vi "Servidor - Fabrica.vi"() -> ()   [LabVIEW 2018]
doc: "Demonstrates how to establish multiple connections and place them in a queue to be serviced. As connections are made, it sends the current date and time via TCP to all Client VIs that connect to it.\n\nThis VI has two parts -- a loop that listens for each client to connect, and a loop that sends the date and time to each connection in the queue.\n\n<B>Note:</B> Use this VI with Multiple Connections - Client 1.vi and Multiple Connections - Client 2.vi."
uses:
  <vilib>/Utility/file.llb/Write Delimited Spreadsheet (string).vi
panel:
  out "Funcionamento:":string
  out "Alertas":u32(colorbox)
  in  "Histórico":i32(listbox)
  out "Thermometro\nForno":dbl(slide) scale=0.0..100.0
  out "Estoque\nProduto Final":dbl(slide) scale=0.0..2500.0
  out "Em Forno?":bool
  out "Misturando?":bool
  out "Solicitação\nMaterial B":dbl
  out "Solicitação\nMaterial A":dbl
  out "Estoque\nMaterial B":dbl(slide) scale=0.0..1200.0
  out "Estoque\nMaterial A":dbl(slide) scale=0.0..1200.0
  out "Mensagem da Produção:":string
  in  "Cliente a Receber os Dados:":string
  out "Cliente - Emissor de Dados:":string
  in  "Temperatura \nProdução [°C]":dbl(slide) scale=0.0..100.0
  out "Produto B":dbl
  in  "Produto A":dbl min=0.0 max=1000.0 step=1.0
  in  "Enviar Produção?":bool
  out "error out":errorcluster
  in  "RESETAR":bool
  in  "Iniciar\nProdução":bool
  in  "empty 3":refnum<k5>[](array[refnum])
  in  "stop":bool
  out "Protocolo de Envio:":string
  out "Conexões":i32
  in  "Porta":u16=6341
  out "IP da Máquina":string
  out "Mensagens":string
  in  "Enviar Todos":bool
  in  "listen halted":bool
  in  "empty":refnum<k5>[](array[refnum])
  # "SERVIDOR - FÁBRICA"
  # "Controle de Produção - Gerência"
  # "Kg"
  # "ON"
  # "ON"
  # "Kg"
  # "OFF"
  # "OFF"
  # "Levantamento de Dados da Produção"
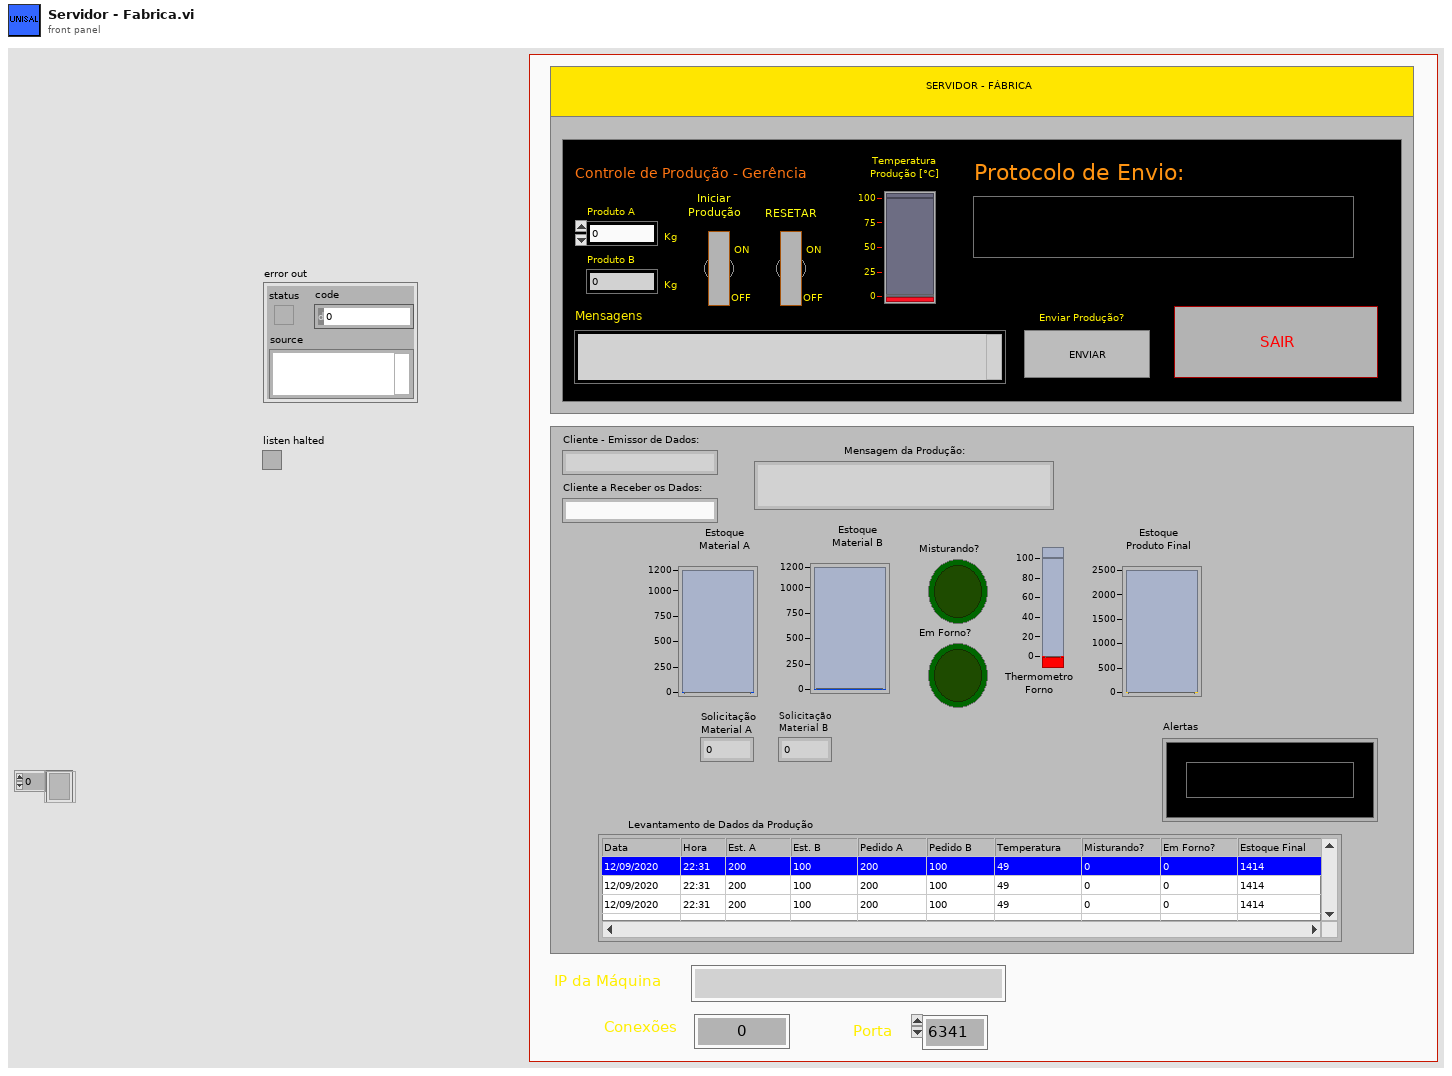
[diagram p1: front panel]
types:
  T1 = enum16{"Standard", "Buffered", "CRLF", "Immediate"}
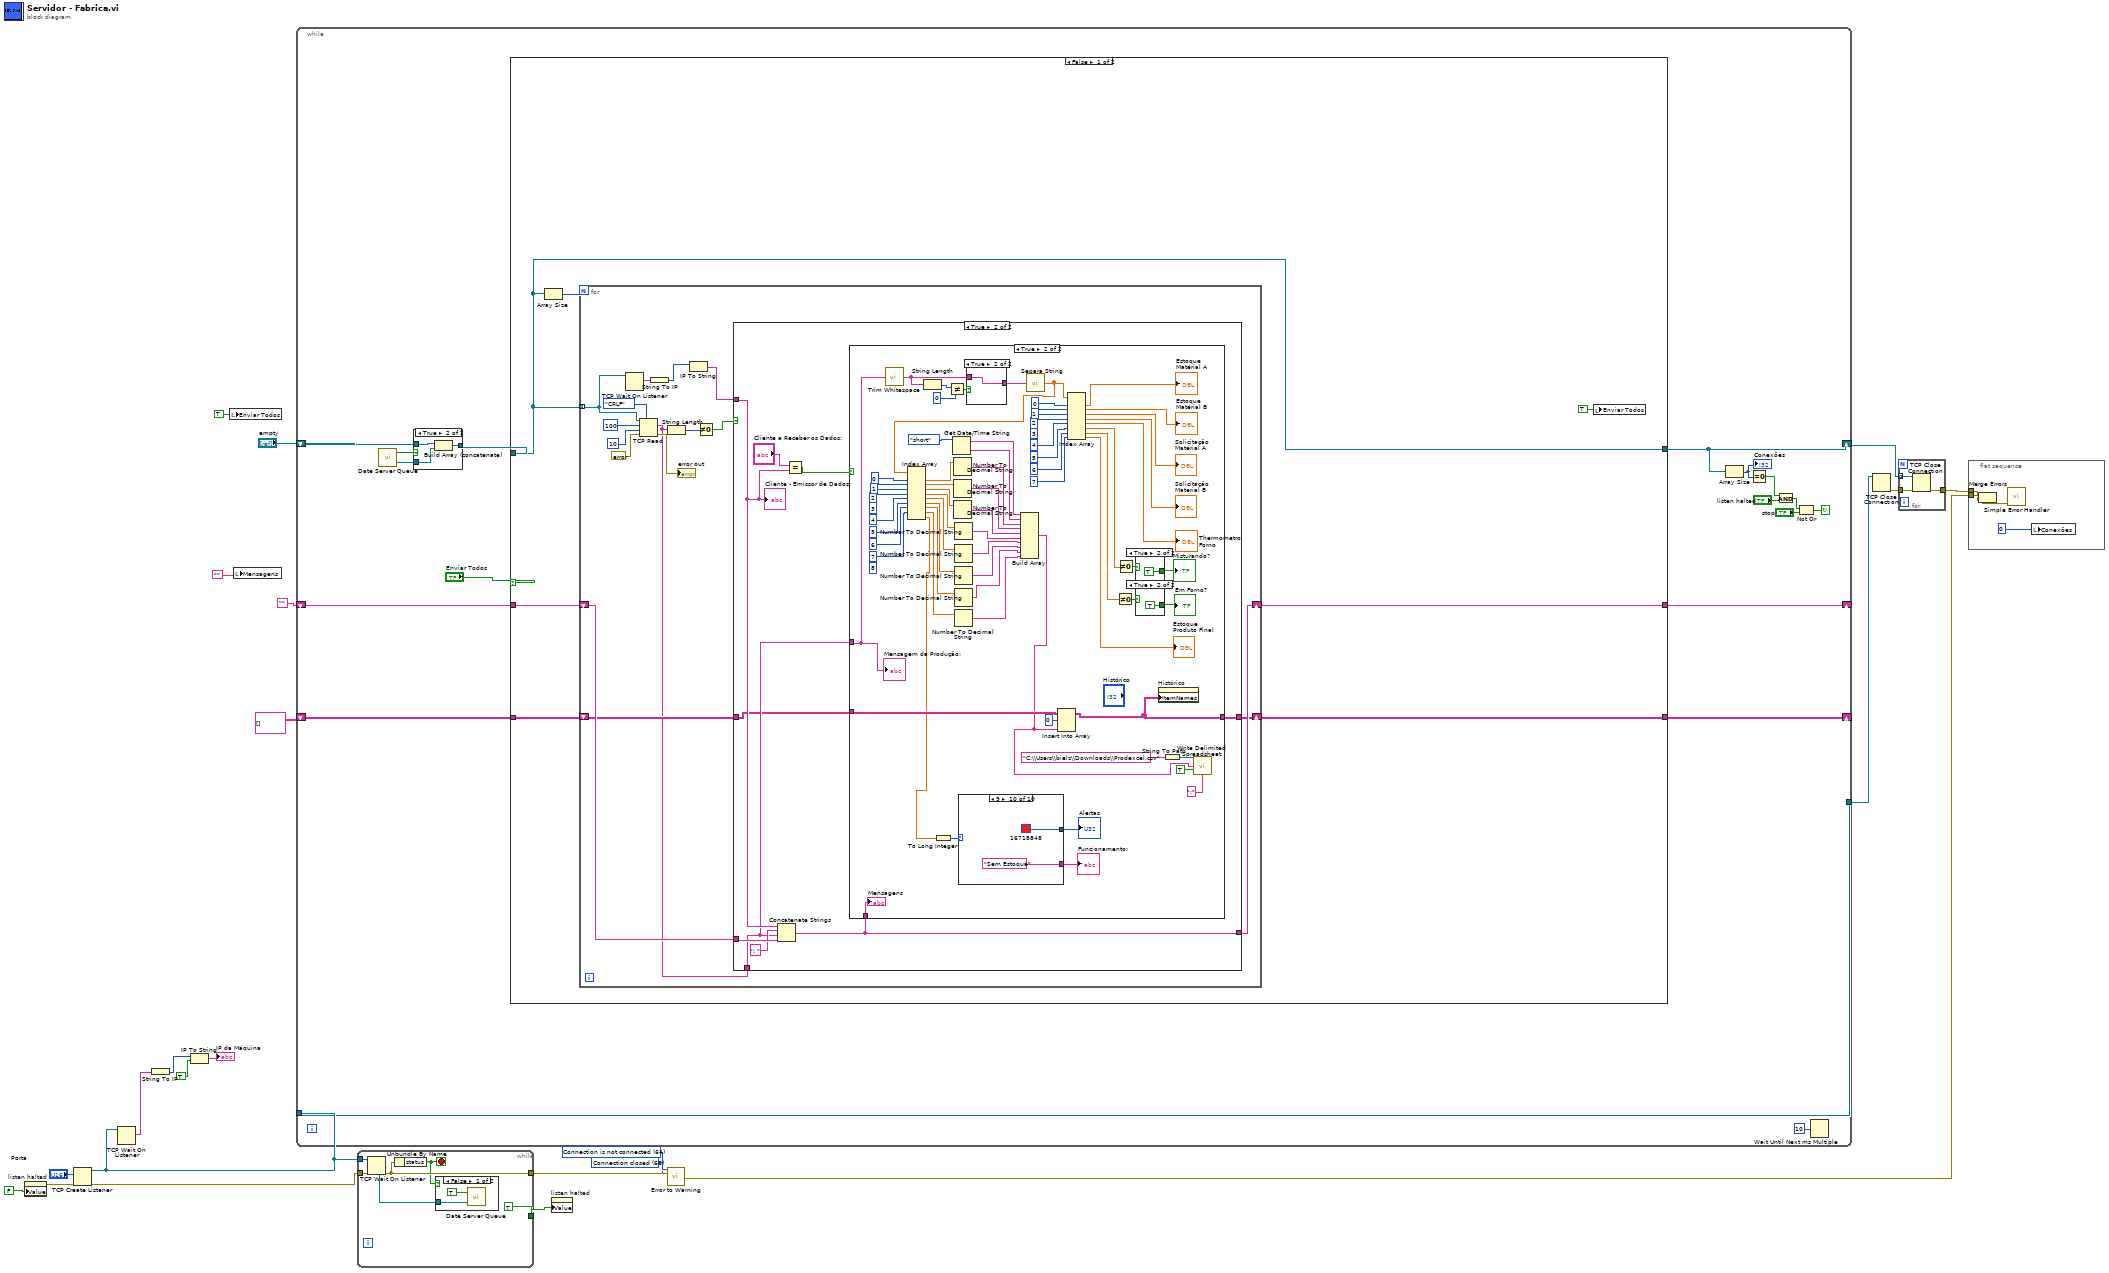
[diagram p0: block diagram]
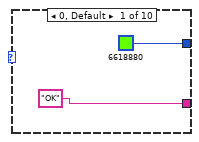
[diagram p4: hidden frame]
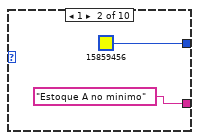
[diagram p5: hidden frame]
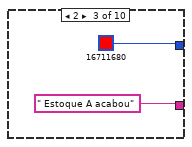
[diagram p6: hidden frame]
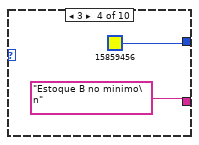
[diagram p7: hidden frame]
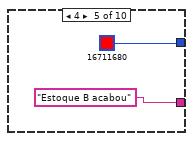
[diagram p8: hidden frame]
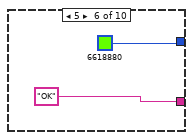
[diagram p9: hidden frame]
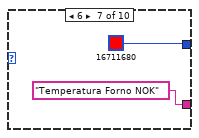
[diagram p10: hidden frame]
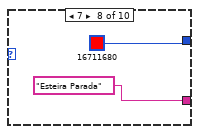
[diagram p11: hidden frame]
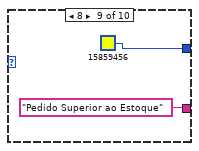
[diagram p12: hidden frame]
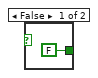
[diagram p13: hidden frame]
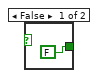
[diagram p14: hidden frame]
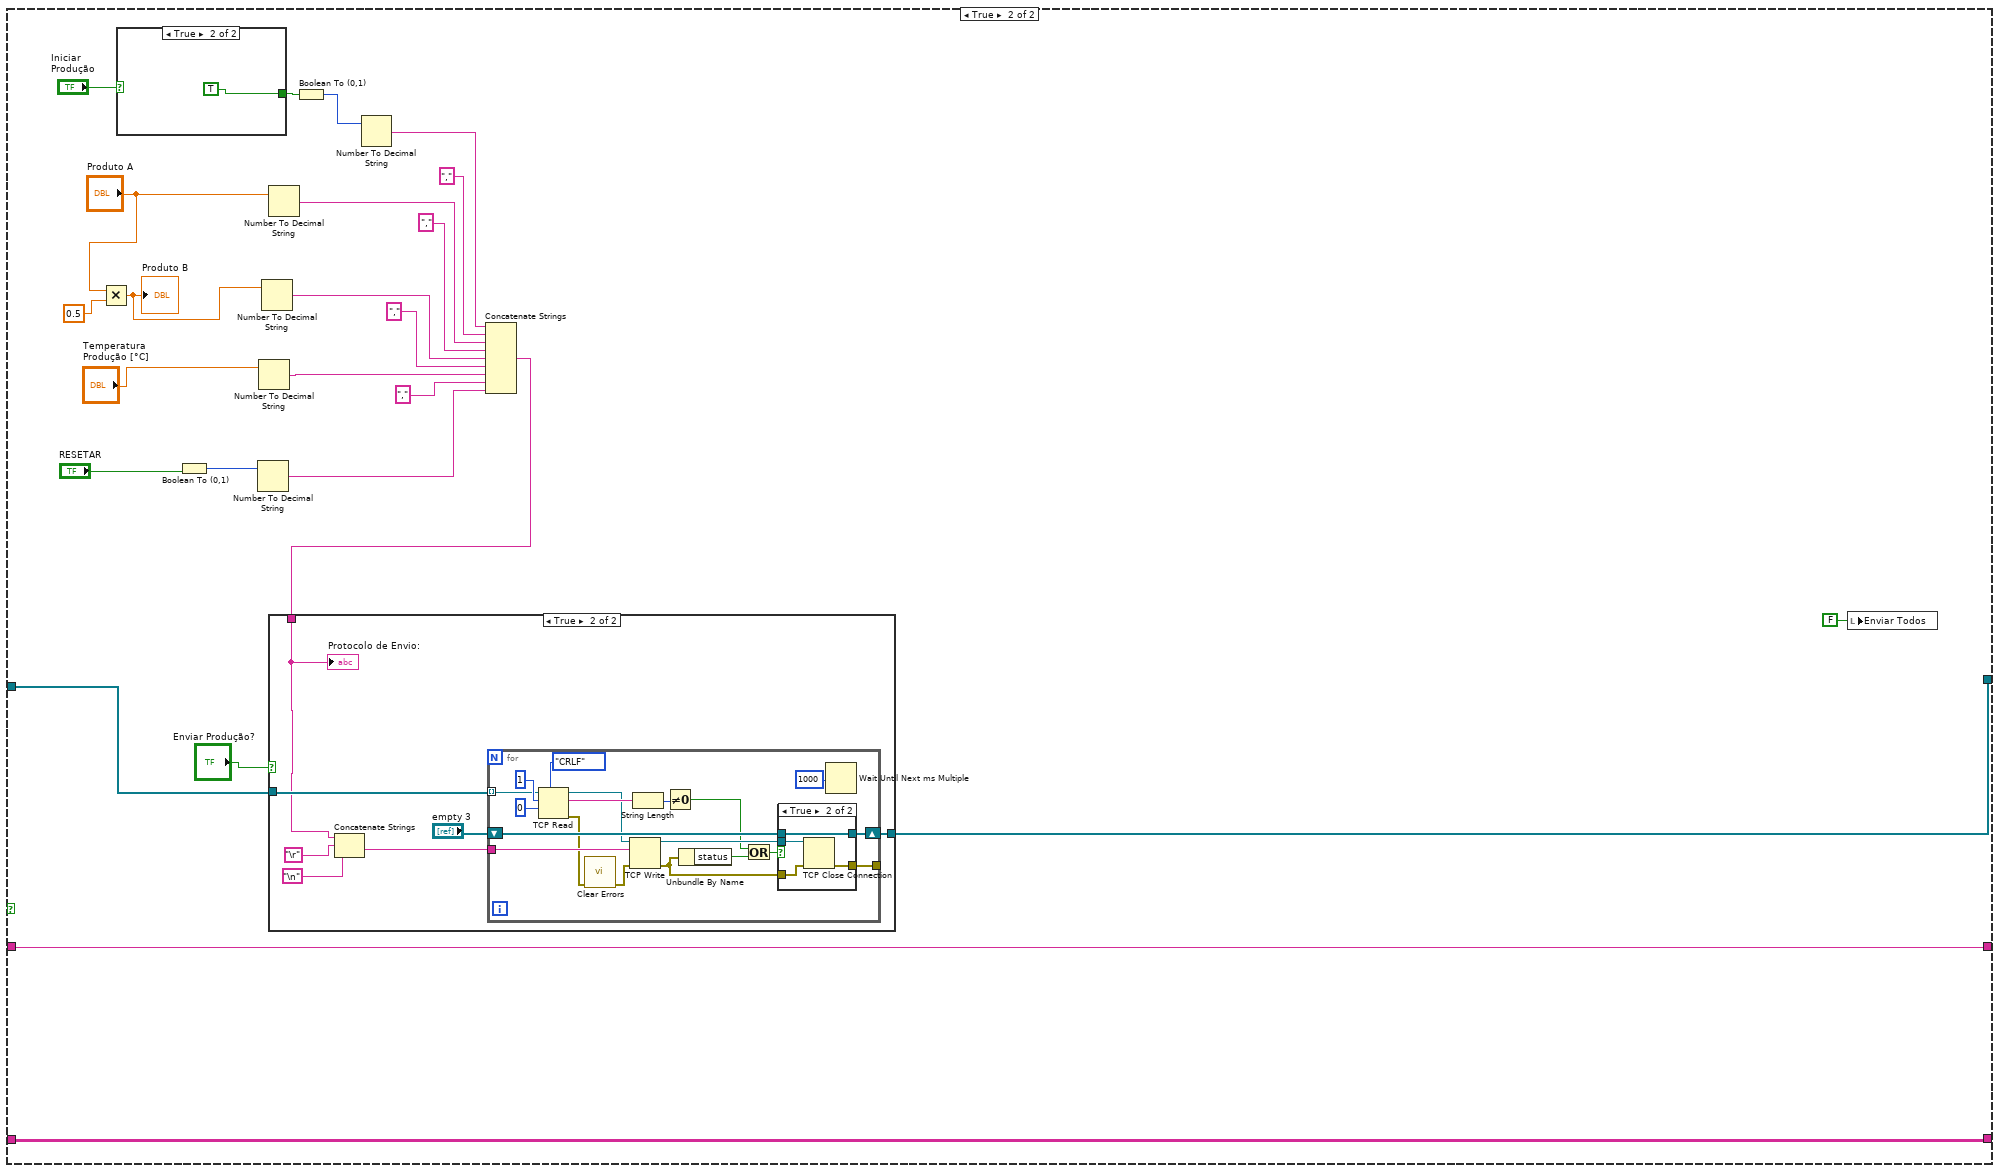
[diagram p16: hidden frame]
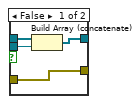
[diagram p18: hidden frame]
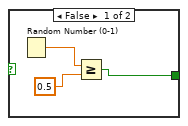
[diagram p19: hidden frame]
diagram:
  w16 = 66 items=["No Error", "Argument Error", "Memory Full", "Out of Zone", "End of File", "File Already Open", "Generic File IO Error", "File Not Found", "File Permission Error", "Disk Full", "Duplicate Path", "Too Many Files Open", "Not Enabled", "Resource File Not Found", "Cannot Add Resource", "Resource Not Found", "Image Not Found", "Image Memory Error", "Pen Does Not Exist", "Config Bad Type", "Config Token Not Found", "Config Parse Error", "Config Memory Error", "Bad External Code Format", "Bad External Code Offset", "External Code Not Present", "Null Window", "Destroy Window Mixup", "Null Menu", "Print Aborted", "Bad Print Record", "Print Driver Error", "Windows Error During Print", "Memory Error During Print", "Print Dialog Error", "Generic Print Error", "Invalid Device Refnum", "Device Not Found", "Device Parameter Error", "Device Unit Error", "Can't Open Device", "Device Call Aborted", "Generic Error", "Cancelled By User", "Object ID Too Low", "Object ID Too High", "Object Not In Heap", "Unknown Heap", "Bad DefProc ID", "DefProc Not In Table", "Message Out Of Range", "Null Method", "Unknown Message", "Manager Call Not Supported", "Bad address", "Connection In progress", "Connection timed out", "Connection is already in progress", "Network attribute not supported", "Network error", "Address in use", "System out of memory", "Connection aborted", "Connection refused", "Connection is not connected", "Connection is already connected", "Connection closed", "Initialize error (interapplication manager)", "Bad occurrence", "Wait on unbound occurrence handler", "Occurrence queue overflow", "Bad path", "Semaphore not signaled", "Unrecognized type (interapplication manager)"] ("2nd Error to Convert")
  w17 = 64 items=["No Error", "Argument Error", "Memory Full", "Out of Zone", "End of File", "File Already Open", "Generic File IO Error", "File Not Found", "File Permission Error", "Disk Full", "Duplicate Path", "Too Many Files Open", "Not Enabled", "Resource File Not Found", "Cannot Add Resource", "Resource Not Found", "Image Not Found", "Image Memory Error", "Pen Does Not Exist", "Config Bad Type", "Config Token Not Found", "Config Parse Error", "Config Memory Error", "Bad External Code Format", "Bad External Code Offset", "External Code Not Present", "Null Window", "Destroy Window Mixup", "Null Menu", "Print Aborted", "Bad Print Record", "Print Driver Error", "Windows Error During Print", "Memory Error During Print", "Print Dialog Error", "Generic Print Error", "Invalid Device Refnum", "Device Not Found", "Device Parameter Error", "Device Unit Error", "Can't Open Device", "Device Call Aborted", "Generic Error", "Cancelled By User", "Object ID Too Low", "Object ID Too High", "Object Not In Heap", "Unknown Heap", "Bad DefProc ID", "DefProc Not In Table", "Message Out Of Range", "Null Method", "Unknown Message", "Manager Call Not Supported", "Bad address", "Connection In progress", "Connection timed out", "Connection is already in progress", "Network attribute not supported", "Network error", "Address in use", "System out of memory", "Connection aborted", "Connection refused", "Connection is not connected", "Connection is already connected", "Connection closed", "Initialize error (interapplication manager)", "Bad occurrence", "Wait on unbound occurrence handler", "Occurrence queue overflow", "Bad path", "Semaphore not signaled", "Unrecognized type (interapplication manager)"] ("1st Error to Convert")
  n1 = property on="listen halted" class="Bool (strict)"("Value"=FALSE) -> (error out=w13:errorcluster)  [unwired: 2 in, 1 out]
  n2 = TCP Create Listener(8:w13, 10:"Porta") -> (0:w21:errorcluster, 3:w8:refnum<k5>)  [unwired: 3 in, 1 out]
  n3 = TCP Wait On Listener(11:w8) -> (2:w7:string)  [unwired: 3 in, 4 out]
  n4 = String To IP(1:w7) -> (0:w6:u32)
  n5 = IP To String(1:TRUE ("dot notation? (F)"), 2:w6) -> (0:→"IP da Máquina":string)
  n6 = local write "Enviar Todos"(TRUE ("Enviar Todos")) -> ()
  n7 = local write "Mensagens"("") -> ()
  n8 = while {
    shift-left: "empty" -> [w39]
    shift-right: [w31] -> w23
    tunnel: w8 -> [w32]
    tunnel: [w32] -> w20
    shift-right: [w27] -> _
    shift-left: "" -> [w28]
    shift-right: [w24] -> _
    shift-left: string[][] [] -> [w25]
    stop <- w34 continue-if-true
    n9 = call <vilib>:"Date Server Queue.vi"() -> ("value"=w41:refnum<k5>, "valid?"=w40:bool)  [unwired: 2 in]
    n10 = case shown="True" w40 {
      tunnel: w41 -> [_ w236]
      tunnel: w39 -> [w233 w235]
      tunnel: [w233 w234] -> w30
      frame False {
      }
      frame True {
        n11 = Build Array (concatenate)(w235, w236) -> (w234:refnum<k5>[])
      }
    }
    n12 = case shown="False" "Enviar Todos" {
      tunnel: w30 -> [w44 w193]
      tunnel: [w44 w192] -> w31
      tunnel: w28 -> [w47 w187]
      tunnel: [w46 w187] -> w27
      tunnel: w25 -> [w43 w169]
      tunnel: [w42 w169] -> w24
      frame False {
        n13 = Array Size(array=w44) -> (size(s)=w45:i32)
        n14 = for {
          N: w45 -> [_]
          tunnel: w44 -> [w53] mode=indexing
          shift-right: [w59] -> w46
          shift-left: w47 -> [w60]
          shift-right: [w50] -> w42
          shift-left: w43 -> [w51]
          n15 = TCP Wait On Listener(11:w53) -> (2:w55:string)  [unwired: 3 in, 4 out]
          n16 = TCP Read(connection ID=w53, bytes to read=100, error in (no error)=errorcluster {"status"=FALSE, "code"=0, "source"=""}, 7:T1."CRLF" ("mode (standard)"), 9:10 ("timeout ms (25000)")) -> (data out=w49:string, error out=→"error out":errorcluster)  [unwired: 1 out]
          n17 = String To IP(1:w55) -> (0:w54:u32)
          n18 = String Length(string=w49) -> (length=w63:i32)
          n19 = IP To String(2:w54) -> (0:w52:string)  [unwired: 1 in]
          n20 = Not Equal To 0?(x=w63) -> (x != 0?=w62:bool)
          n21 = case shown="True" w62 {
            tunnel: w49 -> [_ w70]
            tunnel: w60 -> [w66 w75]
            tunnel: [w66 w71] -> w59
            tunnel: w52 -> [_ w73]
            tunnel: w51 -> [w65 w69]
            tunnel: [w65 w68] -> w50
            frame False {
            }
            frame True {
              n22 = Concatenate Strings(w73, ": ", w70, w75) -> (w71:string)
              n23 = Equal?(x="Cliente a Receber os Dados:", y=w73) -> (x = y?=w67:bool)
              n24 = case shown="True" w67 {
                tunnel: w71 -> [_ w143]
                tunnel: w70 -> [_ w132]
                tunnel: w69 -> [w76 w87]
                tunnel: [w76 w86] -> w68
                frame False {
                }
                frame True {
                  (unwired) 8
                  n25 = call <vilib>:"Trim Whitespace.vi"("string"=w132) -> ("trimmed string"=w135:string)  [unwired: 1 in]
                  n26 = String Length(string=w135) -> (length=w134:i32)
                  n27 = Not Equal?(x=w134, y=0) -> (x != y?=w137:bool)
                  n28 = Get Date/Time String(date format (0)=enum16{"short", "long", "abbreviated"}."short") -> (date string=w98:string, time string=w97:string)  [unwired: 2 in]
                  n29 = case shown="True" w137 {
                    tunnel: [_ w168] -> w136
                    tunnel: w135 -> [_ w168]
                    frame False {
                    }
                    frame True {
                    }
                  }
                  n30 = call "Separa String.vi"("TEXTO DE ENTRADA"=w136) -> ("VETOR DE SAIDA"=w108:dbl[])
                  n31 = Index Array(array=w108, index #1=0 ("index"), index #2=1 ("index"), index #3=2 ("index"), index #4=3 ("index"), index #5=4 ("index"), index #6=5, index #7=6, index #8=7) -> (element #1=w106:dbl, element #2=w105:dbl, element #3=w104:dbl, element #4=w103:dbl, element #5=w102:dbl, element #6=w101:dbl, element #7=w100:dbl, element #8=w99:dbl, element #9=w77:dbl)  [unwired: 1 in]
                  n32 = To Long Integer(number=w77) -> (32bit integer=w78:i32)
                  n33 = Number To Decimal String(number=w106) -> (decimal integer string=w96:string)  [unwired: 1 in]
                  n34 = Number To Decimal String(number=w105) -> (decimal integer string=w95:string)  [unwired: 1 in]
                  n35 = Number To Decimal String(number=w104) -> (decimal integer string=w94:string)  [unwired: 1 in]
                  n36 = Number To Decimal String(number=w103) -> (decimal integer string=w93:string)  [unwired: 1 in]
                  n37 = Number To Decimal String(number=w102) -> (decimal integer string=w92:string)  [unwired: 1 in]
                  n38 = Number To Decimal String(number=w101) -> (decimal integer string=w91:string)  [unwired: 1 in]
                  n39 = Number To Decimal String(number=w100) -> (decimal integer string=w90:string)  [unwired: 1 in]
                  n40 = Number To Decimal String(number=w99) -> (decimal integer string=w89:string)  [unwired: 1 in]
                  n41 = case shown="9" w78 {
                    tunnel: ["OK" "Estoque A no minimo" " Estoque A acabou" "Estoque B no minimo\n" "Estoque B acabou" "OK" "Temperatura Forno NOK" "Esteira Parada" "Pedido Superior ao Estoque" "Sem Estoque"] -> w80
                    tunnel: [u32 6618880 ("Pedido") u32 15859456 ("Pedido") u32 16711680 ("Pedido") u32 15859456 ("Pedido") u32 16711680 ("Pedido") u32 6618880 ("Pedido") u32 16711680 ("Pedido") u32 16711680 ("Pedido") u32 15859456 ("Pedido") u32 16718848 ("Pedido")] -> w79
                    frame 0, Default {
                    }
                    frame 1 {
                    }
                    frame 2 {
                    }
                    frame 3 {
                    }
                    frame 4 {
                    }
                    frame 5 {
                    }
                    frame 6 {
                    }
                    frame 7 {
                    }
                    frame 8 {
                    }
                    frame 9 {
                    }
                  }
                  "Alertas" <- w79
                  "Funcionamento:" <- w80
                  n42 = Build Array(w98, w97, w96, w95, w94, w93, w92, w91, w90, w89) -> (w81:string[])
                  n43 = Insert Into Array(array=w87, index (row)=0 ("index"), new element=w81) -> (w86:string[][])  [unwired: 1 in]
                  n44 = Index Array(array=w108, index #1=0 ("index"), index #2=1 ("index"), index #3=2 ("index"), index #4=3 ("index"), index #5=4 ("index"), index #6=5, index #7=6, index #8=7) -> (element #1=→"Estoque\nMaterial A":dbl, element #2=→"Estoque\nMaterial B":dbl, element #3=→"Solicitação\nMaterial A":dbl, element #4=→"Solicitação\nMaterial B":dbl, element #5=→"Thermometro\nForno":dbl, element #6=w119:dbl, element #7=w118:dbl, element #8=→"Estoque\nProduto Final":dbl)
                  n45 = Not Equal To 0?(x=w118) -> (x != 0?=w124:bool)
                  n46 = Not Equal To 0?(x=w119) -> (x != 0?=w123:bool)
                  n47 = case shown="True" w123 {
                    tunnel: [FALSE TRUE] -> w126
                    frame False {
                    }
                    frame True {
                    }
                  }
                  "Misturando?" <- w126
                  n48 = case shown="True" w124 {
                    tunnel: [FALSE TRUE] -> w125
                    frame False {
                    }
                    frame True {
                    }
                  }
                  "Em Forno?" <- w125
                  n49 = property on="Histórico" class="MCListbox (strict)"("ItemNames"=w86) -> ()  [unwired: 2 in, 2 out]
                  n50 = String To Path(string="C:\\Users\\bielz\\Downloads\\Prodexcel.csv") -> (path=w83:path)
                  n51 = call-poly <vilib>:"Write Delimited Spreadsheet.vi"("file path (dialog if empty)"=w83, "1D data"=w81, "append to file? (new file:F)"=TRUE, "delimiter (\\t)"=";") -> ()  [unwired: 10 in, 2 out]
                  "Mensagens" <- w143
                  "Mensagem da Produção:" <- w132
                }
              }
              "Cliente - Emissor de Dados:" <- w73
            }
          }
        }
        n52 = local write "Enviar Todos"(TRUE ("Enviar Todos")) -> ()
      }
      frame True {
        n53 = Multiply(x="Produto A", y=0.5) -> (x*y=w181:dbl)
        "Produto B" <- w181
        n54 = case shown="True" "Iniciar\nProdução" {
          tunnel: [w229 TRUE] -> w189
          frame False {
            n55 = Random Number (0-1)() -> (number: 0 to 1=w231:dbl)
            n56 = Greater Or Equal?(x=w231, y=0.5) -> (x >= y?=w229:bool)
          }
          frame True {
          }
        }
        n57 = Boolean To (0,1)(Boolean="RESETAR") -> (0, 1=w184:i16)
        n58 = Number To Decimal String(number=w184) -> (decimal integer string=w173:string)  [unwired: 1 in]
        n59 = Number To Decimal String(number="Temperatura \nProdução [°C]") -> (decimal integer string=w185:string)  [unwired: 1 in]
        n60 = Number To Decimal String(number=w181) -> (decimal integer string=w176:string)  [unwired: 1 in]
        n61 = Number To Decimal String(number="Produto A") -> (decimal integer string=w179:string)  [unwired: 1 in]
        n62 = Boolean To (0,1)(Boolean=w189) -> (0, 1=w191:i16)
        n63 = Number To Decimal String(number=w191) -> (decimal integer string=w180:string)  [unwired: 1 in]
        n64 = Concatenate Strings(w180, ",", w179, ",", w176, ",", w185, ",", w173) -> (w170:string)
        n65 = case shown="True" "Enviar Produção?" {
          tunnel: w193 -> [w194 w201]
          tunnel: [w194 w200] -> w192
          tunnel: w170 -> [_ w195]
          frame False {
          }
          frame True {
            n66 = Concatenate Strings(w195, "\r", "\n") -> (w197:string)
            n67 = for {
              tunnel: w201 -> [w210] mode=indexing
              shift-right: [w217] -> w200
              shift-left: "empty 3" -> [w219]
              tunnel: w197 -> [w220]
              tunnel: [w204] -> _
              n68 = TCP Read(connection ID=w210, bytes to read=1, 7:T1."CRLF" ("mode (standard)"), 9:0) -> (connection ID out=w209:refnum<k5>, data out=w214:string, error out=w206:errorcluster)  [unwired: 1 in]
              n69 = call <vilib>:"Clear Errors.vi"("error in (no error)"=w206) -> ("error out"=w205:errorcluster)  [unwired: 5 in, 1 out]
              n70 = TCP Write(connection ID=w209, data in=w220, error in (no error)=w205) -> (connection ID out=w218:refnum<k5>, error out=w207:errorcluster)  [unwired: 1 in, 1 out]
              n71 = String Length(string=w214) -> (length=w213:i32)
              n72 = Not Equal To 0?(x=w213) -> (x != 0?=w211:bool)
              n73 = Unbundle By Name(w207) -> ("status"=w208:bool)
              n74 = Or(x=w211, y=w208) -> (x .or. y?=w212:bool)
              n75 = case shown="True" w212 {
                tunnel: w219 -> [w224 w228]
                tunnel: w218 -> [w223 w227]
                tunnel: [w222 w228] -> w217
                tunnel: w207 -> [w221 w226]
                tunnel: [w221 w225] -> w204
                frame False {
                  n76 = Build Array (concatenate)(w224, w223) -> (w222:refnum<k5>[])
                }
                frame True {
                  n77 = TCP Close Connection(connection ID=w227, error in (no error)=w226) -> (error out=w225:errorcluster)  [unwired: 1 in, 1 out]
                }
              }
              n78 = Wait Until Next ms Multiple(millisecond multiple=u32 1000) -> ()  [unwired: 1 out]
            }
            "Protocolo de Envio:" <- w195
          }
        }
        n79 = local write "Enviar Todos"(FALSE ("Enviar Todos")) -> ()
      }
    }
    n80 = Array Size(array=w31) -> (size(s)=w37:i32)
    "Conexões" <- w37
    n81 = Equal To 0?(x=w37) -> (x = 0?=w38:bool)
    n82 = And(x=w38, y="listen halted") -> (x .and. y?=w35:bool)
    n83 = Not Or(1:"stop", 2:w35) -> (0:w34:bool)
    n84 = Wait Until Next ms Multiple(millisecond multiple=u32 10) -> ()  [unwired: 1 out]
  }
  n85 = while "Listen loop.  Append new connections to a synchronized queue." {
    tunnel: w8 -> [w241]
    tunnel: w21 -> [w242]
    tunnel: [w239] -> w18
    tunnel: [TRUE] -> w19
    stop <- w238 stop-if-true
    n86 = TCP Wait On Listener(8:w242, 11:w241) -> (0:w239:errorcluster, 4:w240:refnum<k5>)  [unwired: 2 in, 3 out]
    n87 = Unbundle By Name(w239) -> ("status"=w238:bool)
    n88 = case shown="False" w238 {
      tunnel: w240 -> [w243 _]
      frame False {
        n89 = call <vilib>:"Date Server Queue.vi"("new value"=w243, "set queue? (F: de-queue)"=TRUE) -> ()  [unwired: 2 out]
      }
      frame True {
      }
    }
  }
  n90 = property on="listen halted" class="Bool (strict)"("Value"=w19) -> ()  [unwired: 2 in, 2 out]
  n91 = call <vilib>:"Error to Warning.vi"("1st Error to Convert"=w17, "2nd Error to Convert"=w16, "error in"=w18) -> ("warning out"=w11:errorcluster)  [unwired: 12 in]
  n92 = TCP Close Connection(connection ID=w20) -> (error out=w12:errorcluster)  [unwired: 2 in, 1 out]
  n93 = for {
    tunnel: w23 -> [w247] mode=indexing
    tunnel: [w246] -> w15
    tunnel: w12 -> [w245]
    n94 = TCP Close Connection(connection ID=w247, error in (no error)=w245) -> (error out=w246:errorcluster)  [unwired: 1 in, 1 out]
  }
  n95 = flat-sequence {
    tunnel: w15 -> [w251]
    tunnel: w11 -> [w249]
    frame #0 {
      n96 = Merge Errors(w251, w249) -> (w250:errorcluster)
      n97 = call <vilib>:"Simple Error Handler.vi"("error in (no error)"=w250) -> ()  [unwired: 4 in, 5 out]
      n98 = local write "Conexões"(0) -> ()
    }
  }
